vi "New Results.vi"(7 "Image Nr.":i32, 8 "error in (no error)":errorcluster, 9 "Results In":refnum<class "Analyze Results Base.lvclass">[](array[class]), 10 "Parameters":refnum<class "Analyze Parameter Base.lvclass">[](array[class]), 11 "Launch IMAQ Display in":refnum<class "HIJ Vision Application.lvclass">) -> (0 "error out":errorcluster, 3 "Launch IMAQ Display out":refnum<class "HIJ Vision Application.lvclass">)   [LabVIEW 2020, in "HIJ Vision Application.lvlib" / "HIJ Vision Application.lvclass"]
uses:
  HIJ Vision Application.lvclass
  Analyze/Results and Overlays/Results Base/Analyze Results Base.lvclass
  Analyze/Analyze Parameter/Analyze Parameter Base/Analyze Parameter Base.lvclass
  HIJ Vision Application.lvclass/HIJ Vision Application.ctl
  Read Child Actor Core.vi
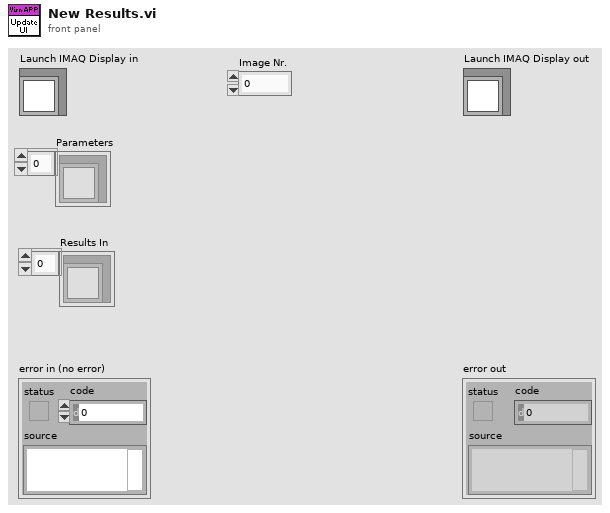
[diagram p1: front panel]
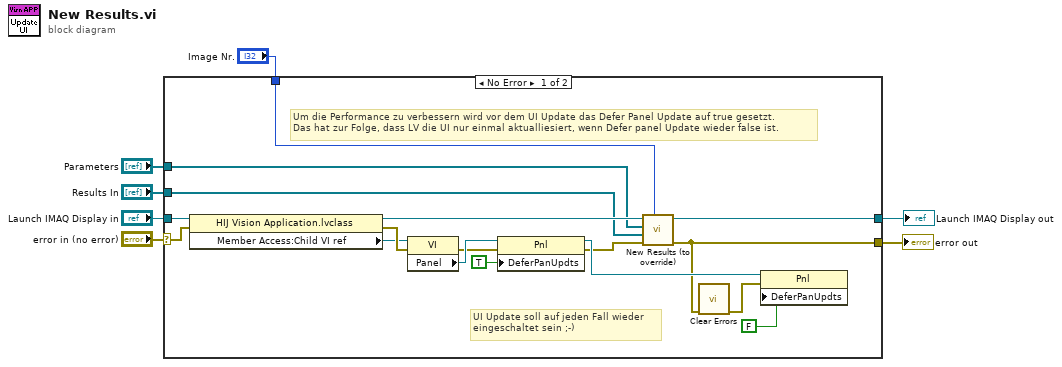
[diagram p0: block diagram]
diagram:
  n1 = case shown="No Error" "error in (no error)" {
    selector: "error in (no error)" -> [w18 w26]
    tunnel: [w10 w26] -> w6
    tunnel: [w14 w25] -> w4
    tunnel: "Launch IMAQ Display in" -> [w24 w25]
    tunnel: "Parameters" -> [w13 _]
    tunnel: "Results In" -> [w12 _]
    tunnel: "Image Nr." -> [w8 _]
    frame No Error {
      # "UI Update soll auf jeden Fall wieder \neingeschaltet sein ;-)"
      # "Um die Performance zu verbessern wird vor dem UI Update das Defer Panel Update auf true gesetzt.\nDas hat zur Folge, dass LV die UI nur einmal aktualliesiert, wenn Defer panel Update wieder false ist."
      n2 = property class="HIJ Vision Application.lvclass"(reference=w24, error in=w18) -> (reference out=w15:refnum<class "HIJ Vision Application.lvclass">, error out=w23:errorcluster, "Member Access:Child VI ref"=w22:refnum<vi>)
      n3 = property class="VI"(reference=w22, error in=w23) -> (error out=w17:errorcluster, "Panel"=w21:refnum<vi>)  [unwired: 1 out]
      n4 = property class="Pnl"(reference=w21, error in=w17, "DeferPanUpdts"=TRUE ("Defer Panel Updates")) -> (reference out=w19:refnum<vi>, error out=w16:errorcluster)
      n5 = call-dynamic "New Results (to override).vi"("Image Nr."=w8, "error in (no error)"=w16, "Results In"=w12, "Parameters"=w13, "Launch IMAQ Display in"=w15) -> ("error out"=w10:errorcluster, "Launch IMAQ Display out"=w14:refnum<class "HIJ Vision Application.lvclass">)  [unwired: 5 in]
      n6 = call <vilib>:"Clear Errors.vi"("error in (no error)"=w10) -> ("error out"=w11:errorcluster)  [unwired: 5 in, 1 out]
      n7 = property class="Pnl"(reference=w19, error in=w11, "DeferPanUpdts"=FALSE ("Defer Panel Updates")) -> ()  [unwired: 2 out]
    }
    frame Error {
    }
  }
  "error out" <- w6
  "Launch IMAQ Display out" <- w4
